vi "Untitled 3.vi"() -> ()   [LabVIEW 2009]
uses:
  <vilib>/rvi/interface/nirviOpenFPGA/nirviOpenFPGA.xnode
  FPGA Bitfiles/Athena Brain.lvproj_FPGA Target 2_vission comm test.vi.lvbitx
  FPGA/IO/vision serial/vission comm test.vi
  <vilib>/FPGAPlugInAG/sbRIO-9642/nirviIntfOpen_sbRIO-9642.vi
  <vilib>/rvi/interface/nirviReadWriteControl/nirviReadWriteControl.xnode
  <vilib>/Utility/error.llb/Error Cluster From Error Code.vi
  <vilib>/rvi/errors/niLvFpgaAdjustHostInterfaceError.vi
  <vilib>/rvi/interface/common/niFpgaNodeNameForErrorReporting.ctl
  <vilib>/rvi/errors/niLvFpgaWhatHappensToTopLevelVI.ctl
  <vilib>/rvi/interface/nirviMethod/nirviMethod.xnode
  <vilib>/rvi/interface/nirviCloseFPGA/nirviCloseFPGA.xnode
  <vilib>/FPGAPlugInAG/sbRIO-9642/nirviIntfClose_sbRIO-9642.vi
  <vilib>/userDefined/High Color/nirio_resource_hc.ctl
  NiRioSrv.dll
panel:
  out "string":string
  in  "stop":bool
  in  "allowed proximity squared":i16=100
  in  "baud rate (9600)":u32=9600
  out "XY Graph":cluster{"Y":dbl[], "Y":dbl[]}[](graph)
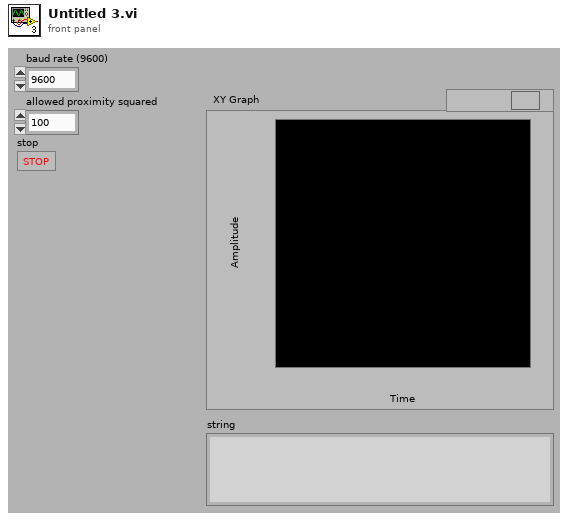
[diagram p1: front panel]
types:
  T1 = typedef "niFpgaNodeNameForErrorReporting.ctl" = enum16{"Open FPGA VI Reference", "Read/Write Control", "Invoke Method: Abort", "Invoke Method: Acknowledge IRQ", "Invoke Method: Download", "Invoke Method: FIFO.Configure", "Invoke Method: FIFO.Read", "Invoke Method: FIFO.Start", "Invoke Method: FIFO.Stop", "Invoke Method: FIFO.Write", "Invoke Method: Reset", "Invoke Method: Run", "Invoke Method: Wait on IRQ", "Close FPGA VI Reference"}
  T2 = typedef "niLvFpgaWhatHappensToTopLevelVI.ctl" = enum16{"top level VI scripted behind XNode", "top level VI inlined behind XNode"}
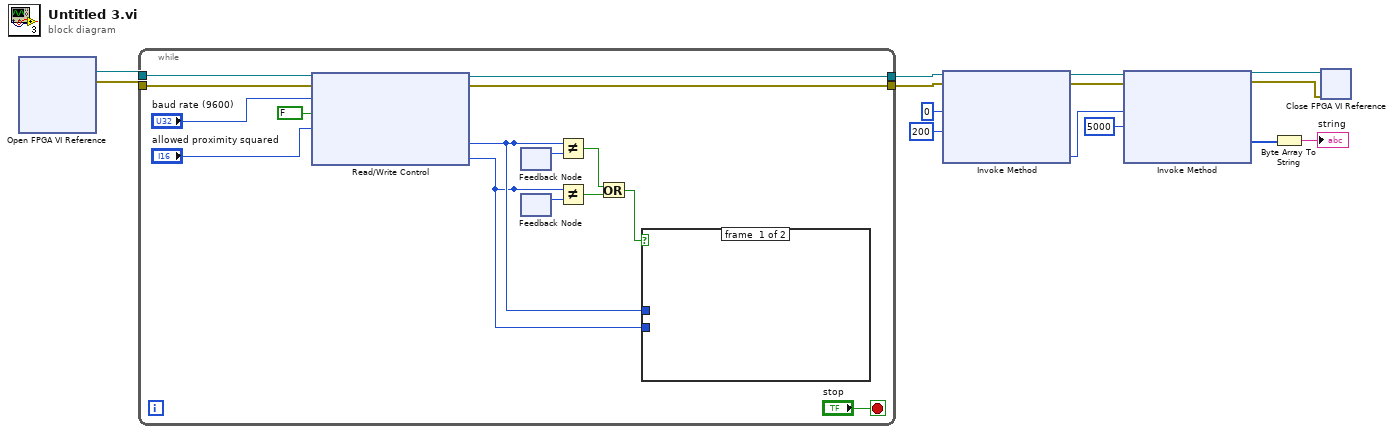
[diagram p0: block diagram]
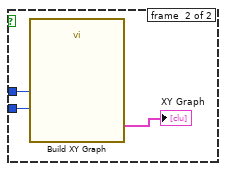
[diagram p2: hidden frame]
diagram:
  n1 = xnode "Open FPGA VI Reference"() -> ("FPGA VI Reference Out"=w14:refnum<k20>, "error out"=w13:errorcluster)  [unwired: 2 in]
  n2 = while {
    tunnel: w14 -> [w29]
    tunnel: w13 -> [w28]
    tunnel: [w27] -> w10
    tunnel: [w19] -> w9
    stop <- "stop" stop-if-true
    n3 = xnode "Read/Write Control"("FPGA VI Reference In"=w29, "error in"=w28, "baud rate (9600)"="baud rate (9600)", "Invert Polarity?"=FALSE, "allowed proximity squared"="allowed proximity squared") -> ("FPGA VI Reference Out"=w27:refnum<k20>, "error out"=w19:errorcluster, "x data"=w22:i16, "y data"=w21:i16)
    n4 = feedback #1() -> (w26:i16)  [unwired: 1 in]
    n5 = feedback #2() -> (w25:i16)  [unwired: 1 in]
    n6 = Not Equal?(x=w22, y=w26) -> (x != y?=w24:bool)
    n7 = Not Equal?(x=w21, y=w25) -> (x != y?=w23:bool)
    n8 = Or(x=w24, y=w23) -> (x .or. y?=w20:bool)
    n9 = case shown="True" w20 {
      tunnel: w22 -> [_ w31]
      tunnel: w21 -> [_ w30]
      frame #0 {
      }
      frame #1 {
        n10 = call "Build XY Graph"("Y Input"=w30, "X Input"=w31) -> ("XY Graph"=→"XY Graph":cluster{"Y":dbl[], "Y":dbl[]}[])  [unwired: 8 in, 1 out]
      }
    }
  }
  n11 = xnode "Invoke Method"("FPGA VI Reference In"=w10, "error in"=w9, "Number of Elements"=u32 0, "Timeout (ms)"=200) -> ("FPGA VI Reference Out"=w8:refnum<k20>, "error out"=w7:errorcluster, "Elements Remaining"=w4:u32)  [unwired: 1 out]
  n12 = xnode "Invoke Method"("FPGA VI Reference In"=w8, "error in"=w7, "Number of Elements"=w4, "Timeout (ms)"=5000) -> ("FPGA VI Reference Out"=w12:refnum<k20>, "error out"=w11:errorcluster, "Data"=w2:u8[])  [unwired: 1 out]
  n13 = Byte Array To String(unsigned byte array=w2) -> (string=→"string":string)
  n14 = xnode "Close FPGA VI Reference"("FPGA VI Reference In"=w12, "error in"=w11) -> ()  [unwired: 1 out]
